vi "Set Data Server Options.vi"(6 "launch data viewer":bool, 8 "error in":errorcluster, 9 "data server frequency (Hz)":dbl(ring)=10.0 items=["0.5 Hz"=0.5, "1.0 Hz"=1.0, "2.0 Hz"=2.0, "2.5 Hz"=2.5, "4.0 Hz"=4.0, "5.0 Hz"=5.0, "8.0 Hz"=8.0, "10.0 Hz"=10.0, "12.5 Hz"=12.5, "20.0 Hz"=20.0, "25.0 Hz"=25.0, "40.0 Hz"=40.0, "50.0 Hz"=50.0, "100.0 Hz"=100.0], 10 "enable data server":bool, 11 "data sharing framework custom device in":T1 format="%.0x") -> (0 "error out":errorcluster, 1 "coerced data server frequency (Hz)":dbl, 3 "data sharing framework custom device out":T1 format="%.0x")   [LabVIEW 2020, in "Data Sharing Framework Custom Device Scripting.lvlib"]
doc: "Writes the <b>data server enabled</b>, <b>data server frequency (Hz)</b>, and <b>launch data viewer</b> options. Use these options to configure a data server and viewer that monitor the data buffer."
uses:
  Data Sharing Framework Custom Device Scripting.lvlib
  <vilib>/NI VeriStand/Custom Device API/Custom Device Item Ref.ctl
  DSF Shared.lvlib
  <vilib>/NI VeriStand/Custom Device API/Custom Device API.lvlib
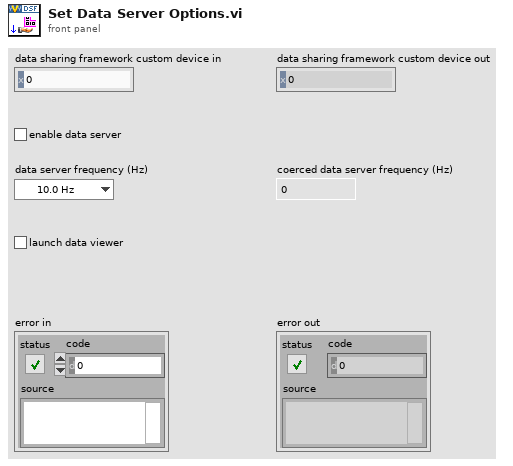
[diagram p1: front panel]
types:
  T1 = typedef "Custom Device API.lvlib/Custom Device Item Ref.ctl" = u64
  T2 = typedef "DSF Core.lvlibp/Framework.lvclass/Framework Options.ctl" = cluster{"FIFO Options":T3, "Thread Options":T4, "Plugin Options":T5, "Performance Options":T6, "Data Server Options":T7}
  T3 = typedef "DSF Core.lvlibp/Framework.lvclass/DSF FIFO Options.ctl" = cluster{"Infinite Timeouts":bool}
  T4 = typedef "DSF Core.lvlibp/Thread.lvclass/Thread Options.ctl" = cluster{"Show FP On Call":bool, "Close FP After Call":bool, "Allow Debugging":bool}
  T5 = typedef "DSF Core.lvlibp/Framework.lvclass/DSF Plugin Options.ctl" = cluster{"Default Components":bool}
  T6 = typedef "DSF Core.lvlibp/DSF Performance Options.ctl" = cluster{"Measure Period":bool, "Measure Rx/Tx Duration":bool}
  T7 = typedef "DSF Core.lvlibp/Framework.lvclass/Data Server Options.ctl" = cluster{"Enable Data Server":bool, "Period":u32}
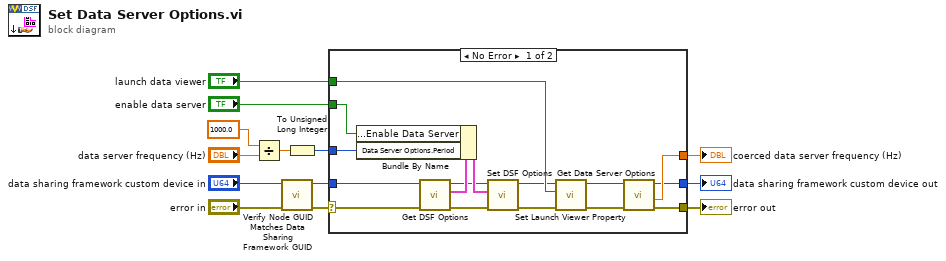
[diagram p0: block diagram]
diagram:
  n1 = Divide(x=1000.0 ("y"), y="data server frequency (Hz)") -> (x/y=w12:dbl)
  n2 = call "Verify Node GUID Matches Data Sharing Framework GUID.vi"("error in"="error in", "data sharing framework custom device in"="data sharing framework custom device in") -> ("error out"=w5:errorcluster, "data sharing framework custom device out"=w4:T1)  [unwired: 8 in]
  n3 = To Unsigned Long Integer(number=w12) -> (unsigned 32bit integer=w11:u32)
  n4 = case shown="No Error" w5 {
    selector: w5 -> [w20 w31]
    tunnel: w11 -> [w28 _]
    tunnel: "enable data server" -> [w24 _]
    tunnel: "launch data viewer" -> [w23 _]
    tunnel: w4 -> [w19 w30]
    tunnel: [w18 w31] -> w3
    tunnel: [w17 _] -> w2
    tunnel: [w16 w30] -> w1
    frame No Error {
      n5 = call "Get DSF Options.vi"("error in (no error)"=w20, "Item Ref in"=w19) -> ("error out"=w29:errorcluster, "options"=w27:T2, "Item Ref out"=w25:T1)  [unwired: 7 in]
      n6 = Bundle By Name(cluster=w27, "Data Server Options.Enable Data Server"=w24, "Data Server Options.Period"=w28) -> (w26:T2)
      n7 = call "Set DSF Options.vi"("error in (no error)"=w29, "options"=w26, "Item Ref in"=w25) -> ("error out"=w21:errorcluster, "Item Ref out"=w22:T1)  [unwired: 7 in]
      n8 = call "Set Launch Viewer Property.vi"("error in (no error)"=w21, "launch viewer"=w23, "Item Ref in"=w22) -> ("error out"=w14:errorcluster, "Item Ref out"=w15:T1)  [unwired: 7 in]
      n9 = call "Get Data Server Options.vi"("error in"=w14, "data sharing framework custom device in"=w15) -> ("error out"=w18:errorcluster, "data server frequency (Hz)"=w17:dbl, "data sharing framework custom device out"=w16:T1)  [unwired: 5 in, 2 out]
    }
    frame Error {
    }
  }
  "data sharing framework custom device out" <- w1
  "error out" <- w3
  "coerced data server frequency (Hz)" <- w2
